vi "UTILITY JKI Loop Timer.vi"(4 "PID gains":T2={"proportional gain (Kc)"=0.1, "integral time (Ti, min)"=0.01, "derivative time (Td, min)"=0.0} {"derivative time (Td, min)" format="%.3f"; "integral time (Ti, min)" format="%.3f"; "proportional gain (Kc)" format="%.3f"}, 6 "Use Fuzzy Logic":bool, 7 "Initialize Rate":bool, 9 "Min Setpoint":T1=0.2 format="%.2f", 10 "K(0.3)":dbl=0.3 format="%#_13g", 11 "Scan Rate (Seconds)":dbl) -> (2 "Rate":dbl, 3 "New Time":dbl)   [LabVIEW 2018]
uses:
  Custom Pallet Controls/Custom Pallet DBL.ctl
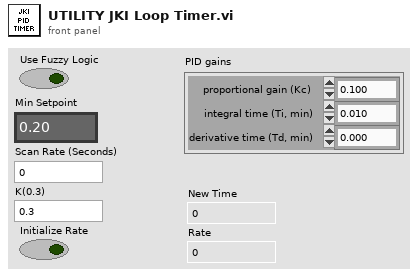
[diagram p1: front panel]
types:
  T1 = typedef "Custom Pallet DBL.ctl" = dbl
  T2 = cluster{"proportional gain (Kc)":dbl, "integral time (Ti, min)":dbl, "derivative time (Td, min)":dbl}
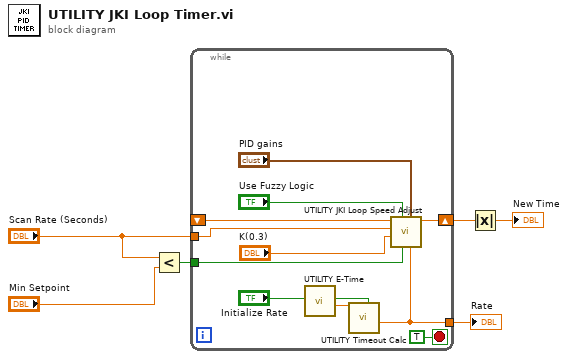
[diagram p0: block diagram]
diagram:
  n1 = Less?(x="Scan Rate (Seconds)", y="Min Setpoint") -> (x < y?=w3:bool)
  n2 = while {
    shift-right: [w12] -> w1
    shift-left: _ -> [w16]
    tunnel: "Scan Rate (Seconds)" -> [w10]
    tunnel: [w11] -> w6
    tunnel: w3 -> [w13]
    stop <- TRUE stop-if-true
    n3 = call "UTILITY E-Time.vi"() -> ("Elapsed Time (sec)"=w17:dbl)  [unwired: 9 in, 2 out]
    n4 = call "UTILITY Timeout Calc.vi"("Initialize Rate"="Initialize Rate", "Timer"=w17) -> ("Rate"=w11:dbl)  [unwired: 8 in, 1 out]
    n5 = call "UTILITY JKI Loop Speed Adjust.vi"("Current Rate"=w11, "PID gains"="PID gains", "Scan Rate Less Than 0.2s"=w13, "Use Fuzzy Logic"="Use Fuzzy Logic", "K(7) - Adjustment Factor"="K(0.3)", "Scan Rate Target"=w10, "Previous Value"=w16) -> ("New Time"=w12:dbl)  [unwired: 4 in]
  }
  "Rate" <- w6
  n6 = Absolute Value(x=w1) -> (abs(x)=→"New Time":dbl)
